vi "Decrypt.vi"(7 "Padding Mode":T1=enum."OaepSHA512", 8 "error in (no error)":errorcluster, 10 "Encrypted data in":u8[](array[numeric]), 11 "CngKey in":refnum<k24>) -> (0 "error out":errorcluster, 2 "Raw data out":u8[](array[numeric]), 3 "CngKey out":refnum<k24>)   [LabVIEW 2021, in "dotNET Crypto Asymmetric Encryption.lvlib"]
doc: "Decrypt RSA-encrypted data using the private key."
uses:
  dotNET Crypto Asymmetric Encryption.lvlib
  RSAEncryptionPadding.ctl
  System.Core
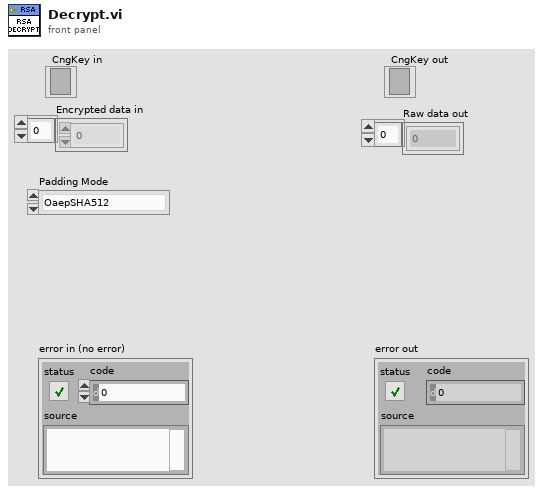
[diagram p1: front panel]
types:
  T1 = typedef "dotNET Crypto Asymmetric Encryption.lvlib/RSAEncryptionPadding.ctl" = enum16{"OaepSHA1", "OaepSHA256", "OaepSHA384", "OaepSHA512", "Pkcs1"}
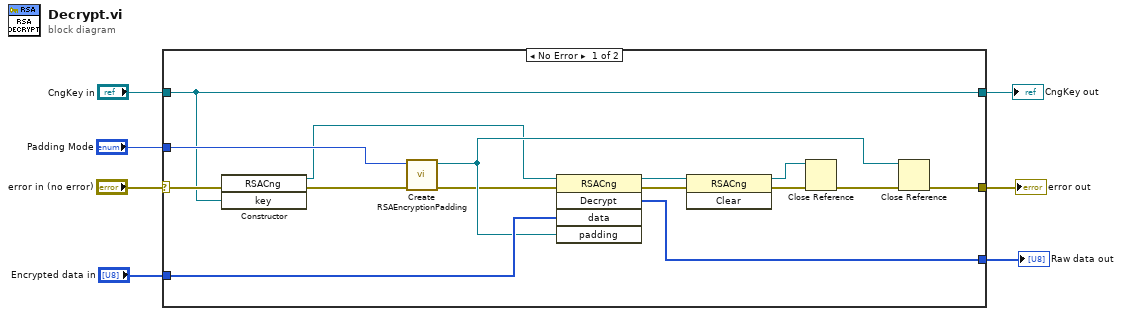
[diagram p0: block diagram]
diagram:
  n1 = case shown="No Error" "error in (no error)" {
    selector: "error in (no error)" -> [w9 w24]
    tunnel: "Encrypted data in" -> [w22 _]
    tunnel: [w21 _] -> w6
    tunnel: "Padding Mode" -> [w14 _]
    tunnel: [w10 w24] -> w4
    tunnel: "CngKey in" -> [w8 w23]
    tunnel: [w8 w23] -> w1
    frame No Error {
      n2 = constructor class="RSACng"(error in=w9, "key"=w8) -> (reference out=w11:refnum<k24>, error out=w12:errorcluster)  [unwired: 2 in, 2 out]
      n3 = call "Create RSAEncryptionPadding.vi"("error in (no error)"=w12, "Padding Mode"=w14) -> ("error out"=w13:errorcluster, "RSAEncryptionPadding"=w15:refnum<k24>)  [unwired: 8 in]
      n4 = invoke class="RSACng" method="Decrypt"(reference=w11, error in=w13, "data"=w22, "padding"=w15) -> (reference out=w19:refnum<k24>, error out=w20:errorcluster, "Decrypt"=w21:u8[])  [unwired: 1 in, 2 out]
      n5 = invoke class="RSACng" method="Clear"(reference=w19, error in=w20) -> (reference out=w17:refnum<k24>, error out=w16:errorcluster)  [unwired: 1 in, 1 out]
      n6 = Close Reference(reference=w17, error in (no error)=w16) -> (error out=w18:errorcluster)
      n7 = Close Reference(reference=w15, error in (no error)=w18) -> (error out=w10:errorcluster)
    }
    frame Error {
    }
  }
  "error out" <- w4
  "Raw data out" <- w6
  "CngKey out" <- w1
